vi "Stop Core.vi"(10 "final error code":i32, 11 "Actor wUI in":refnum<class "Actor wUI.lvclass">) -> (3 "Actor wUI out":refnum<class "Actor wUI.lvclass">)   [LabVIEW 2017, in "Framework.lvlib" / "Actor wUI.lvclass"]
doc: "(<B>Filename</B>: Actor Framework.lvlib:Actor.lvclass:Stop Core.vi)\n\nDefines what the actor does before it stops. Use the <B>final error code</B> input to determine whether the actor shut down in response to an error.\n\nBy default, this method does nothing. A descendant class may override it to define behavior, such as shutting down any processes the actor initiated in its override of the Actor Core method."
uses:
  Actor wUI.lvclass
  Actor wUI.lvclass/Actor wUI.ctl
  <vilib>/ActorFramework/Actor/Actor.lvclass
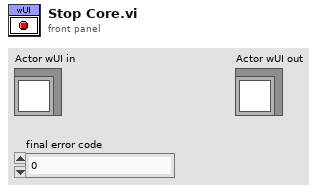
[diagram p1: front panel]
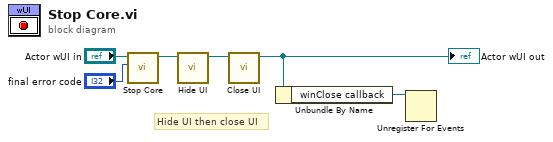
[diagram p0: block diagram]
diagram:
  # "Hide UI then close UI"
  n1 = call-parent "Stop Core.vi"("final error code"="final error code", "Actor in"="Actor wUI in") -> ("Actor out"=w3:refnum<class "Actor wUI.lvclass">)  [unwired: 9 in]
  n2 = call "Hide UI.vi"("Actor wUI in"=w3) -> ("Actor wUI out"=w4:refnum<class "Actor wUI.lvclass">)  [unwired: 9 in, 1 out]
  n3 = call "Close UI.vi"("Actor wUI in"=w4) -> ("Actor wUI out"=w2:refnum<class "Actor wUI.lvclass">)  [unwired: 9 in, 1 out]
  "Actor wUI out" <- w2
  n4 = Unbundle By Name(w2) -> ("winClose callback"=w1:refnum<k27>)
  n5 = Unregister For Events(event registration refnum=w1) -> ()  [unwired: 1 in, 1 out]
